vi "NearFiledCamSetTrigger.vi"(3 "错误输入（无错误）":errorcluster, 5 "触发模式":enum16{"连续触发", "外部触发1", "外部触发2"}(ring)) -> (0 "错误输出":errorcluster)   [LabVIEW 2018]
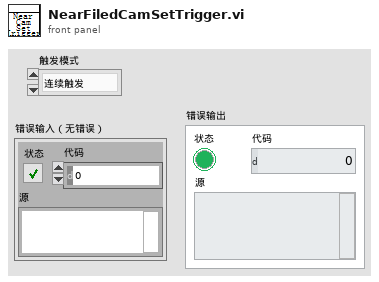
[diagram p1: front panel]
types:
  T1 = typedef "IMAQ Image.ctl" = refnum<image>
  T2 = cluster{"示波器":cluster{"Channel (0:Channel 1)":enum16{"Channel 1", "Channel 2", "Channel 3", "Channel 4"}, "电压范围":dbl, "触发电压":dbl, "时间范围":dbl, " 示波器VISA":refnum<visa-resource-name>, "时间范围 标签":u64, "电压范围 标签":u64, "触发电压 标签":u64, "输入阻抗/Ω":u64, "示波器类型":bool}, "光谱仪":cluster{"SpecDataReference":refnum<queue>, "grating center":dbl, "Exposure Time (s)":dbl, "是否进行详细设置":bool, " 开始通信检查":bool, "通信成功？":bool, "波长":dbl, "LightField Automation out":refnum<class "LightField Automation.lvclass">}, " 近场相机":cluster{"曝光时间/us":dbl, "IP 地址":string, "ImageData":T1, " 曝光最大":i32, " 曝光最小":i32, "Camera Source":refnum<k21>, "近场X范围":dbl, "近场Y范围":dbl, "单个像元大小/um":dbl, "相机距离原点位置":dbl[], "是否测量发散角":bool, "光束类型(发散T)":bool, "聚焦透镜焦距mm":dbl}, " 偏振仪":cluster{"电压范围":u64, "触发电压":u64, "时间范围":u64, "波长范围":enum16{"可见光 400-700nm", "近红外 700-1100nm"}, "可见光偏振测量仪VISA":refnum<visa-resource-name>, "近红外偏振测量仪VISA":refnum<visa-resource-name>}, " 功率计":cluster{"通道":enum16{"Channel 1", "Channel 2"}, "工作波长":u32, "单位":u64, "时间范围":u64, "IP地址":string, "端口":u32, "是否需要散射片":bool}, "能量计":cluster{"通道":enum16{"Channel 1", "Channel 2"}, "工作波长":u32, "单位":u64, "时间范围":u64, "IP地址":string, "端口":u32, "能量计量程":enum16{"200uJ", "20uJ", "2uJ", "200nJ"}}, "电机":cluster{"Channel (0:Channel 1)":enum16{"Channel 1", "Channel 2", "Channel 3", "Channel 4"}, "电压范围":u64, "触发电压":u64, "时间范围":u64}, " 远场相机":cluster{"曝光时间":i32, "IP 地址":string, "ImageData":T1, "  增益最大":i32, "  增益最小":i32, " 曝光最大":i32, " 曝光最小":i32, "ImageData B":T1, "是否远场测量":bool}}
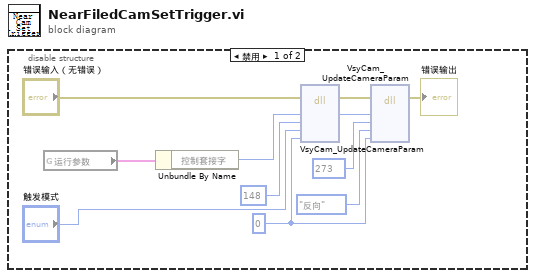
[diagram p0: block diagram]
diagram:
  n1 = disable-structure shown="禁用" {
    frame Disabled {
      w5 = 0 ("ack")
      n2 = global read "参数.vi" "运行参数"() -> (w3:T2)
      n3 = Unbundle By Name(w3) -> ("控制套接字"=w2:i32)
      n4 = dll-call lib="PTH2^abs I航天测量驱动相机驱动LabView2014Demo_V1.0.8\nLabView14Demo\nVsyCam.dll" fn="VsyCam_UpdateCameraParam"(error in="错误输入（无错误）", "sockFd"=w2, "command"=148, "value"="触发模式", "ack"=w5) -> (error out=w10:errorcluster, "sockFd"=w1:i32)  [unwired: 6 in, 1 out]
      n5 = dll-call lib="PTH2^abs I航天测量驱动相机驱动LabView2014Demo_V1.0.8\nLabView14Demo\nVsyCam.dll" fn="VsyCam_UpdateCameraParam"(error in=w10, "sockFd"=w1, "command"=273, "value"=enum16{"同向", "反向"}."反向" ("触发模式"), "ack"=w5) -> (error out=→"错误输出":errorcluster)  [unwired: 7 in, 1 out]
    }
    frame Enabled {
    }
  }
